vi "OA Acc.vi"(7 "SlaveID":u8=1, 8 "error in (no error)":errorcluster, 11 ".NET Refnum in":refnum<k24>) -> (0 "error out":errorcluster, 2 "OA Acc":u16[](array[numeric]), 3 "reference out":refnum<k24>)   [LabVIEW 2017]
uses:
  DLL/Modbus.dll
panel:
  out "x-y":u32
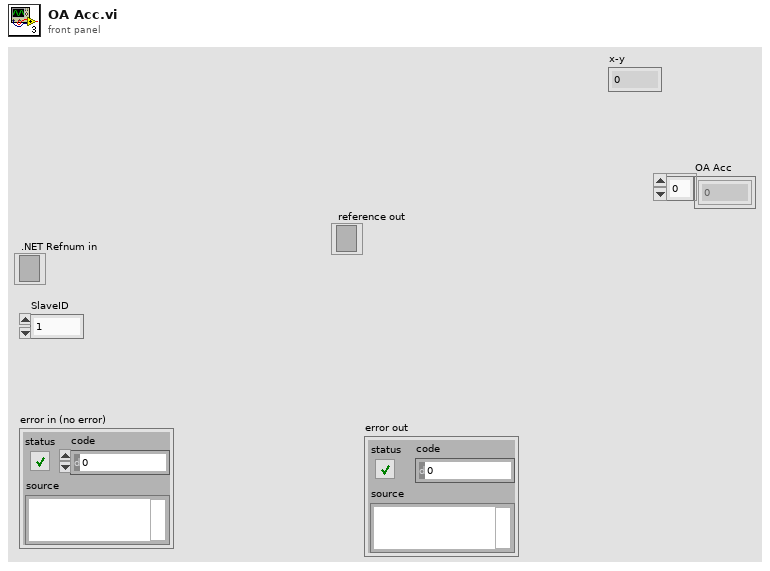
[diagram p1: front panel]
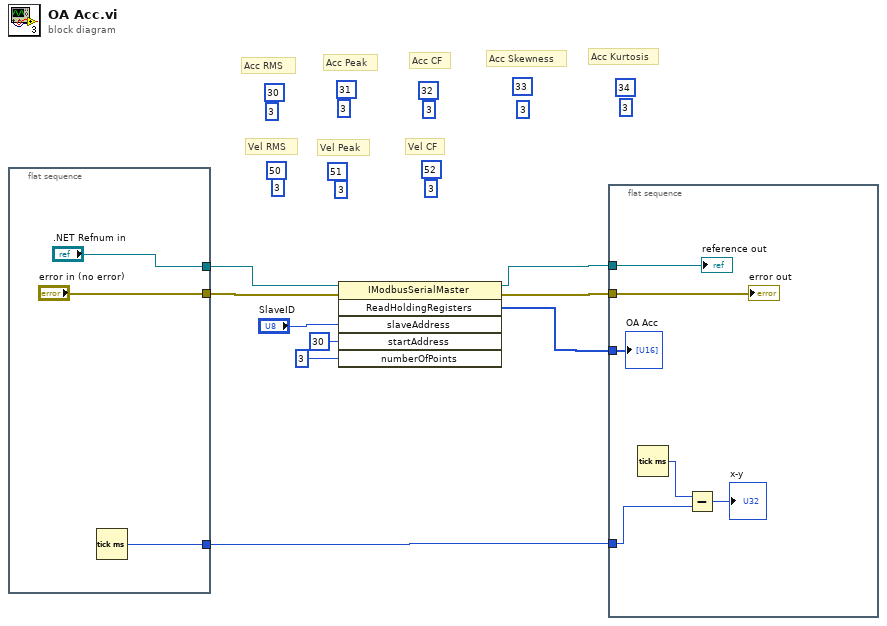
[diagram p0: block diagram]
diagram:
  (unwired) u16 3 ("numberOfPoints")
  (unwired) u16 3 ("numberOfPoints")
  (unwired) u16 52 ("startAddress")
  (unwired) u16 51 ("startAddress")
  (unwired) u16 3 ("numberOfPoints")
  (unwired) u16 3 ("numberOfPoints")
  (unwired) u16 3 ("numberOfPoints")
  (unwired) u16 50 ("startAddress")
  (unwired) u16 34 ("startAddress")
  (unwired) u16 33 ("startAddress")
  (unwired) u16 3 ("numberOfPoints")
  (unwired) u16 32 ("startAddress")
  (unwired) u16 3 ("numberOfPoints")
  (unwired) u16 31 ("startAddress")
  (unwired) u16 3 ("numberOfPoints")
  (unwired) u16 30 ("startAddress")
  # "Vel CF"
  # "Vel Peak"
  # "Vel RMS"
  # "Acc Kurtosis"
  # "Acc Skewness"
  # "Acc CF"
  # "Acc Peak"
  # "Acc RMS"
  n1 = flat-sequence {
    tunnel: ["error in (no error)"] -> w9
    tunnel: [".NET Refnum in"] -> w8
    tunnel: [w10] -> w4
    frame #0 {
      n2 = Tick Count (ms)() -> (millisecond timer value=w10:u32)
    }
  }
  n3 = invoke class="IModbusSerialMaster" method="ReadHoldingRegisters"(reference=w8, error in=w9, "slaveAddress"="SlaveID", "startAddress"=u16 30, "numberOfPoints"=u16 3) -> (reference out=w6:refnum<k24>, error out=w7:errorcluster, "ReadHoldingRegisters"=w5:u16[])  [unwired: 1 in, 3 out]
  n4 = flat-sequence {
    tunnel: w7 -> [w18]
    tunnel: w6 -> [w17]
    tunnel: w5 -> [w13]
    tunnel: w4 -> [w15]
    frame #0 {
      n5 = Tick Count (ms)() -> (millisecond timer value=w16:u32)
      n6 = Subtract(x=w16, y=w15) -> (x-y=→"x-y":u32)
      "error out" <- w18
      "reference out" <- w17
      "OA Acc" <- w13
    }
  }
